vi "reseter.vi"(7 "Mode":enum16{"Init", "Set", "Get"}(ring)=enum."Get", 8 "Error In":errorcluster, 11 "Value":bool) -> (0 "Error Out":errorcluster, 3 "Value":bool)   [LabVIEW 2016]
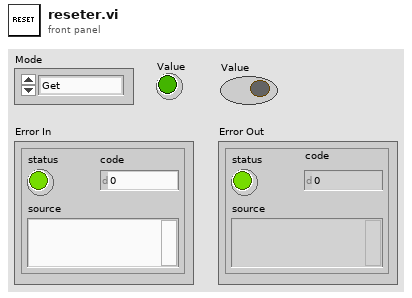
[diagram p1: front panel]
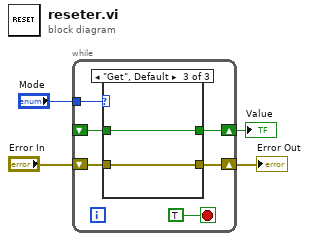
[diagram p0: block diagram]
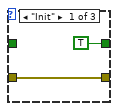
[diagram p2: hidden frame]
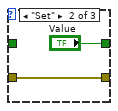
[diagram p3: hidden frame]
diagram:
  n1 = while {
    tunnel: "Mode" -> [w9]
    shift-right: [w7] -> w2
    shift-left: "Error In" -> [w8]
    shift-right: [w6] -> w1
    shift-left: _ -> [w5]
    stop <- TRUE stop-if-true
    n2 = case shown="\"Get\", Default" w9 {
      tunnel: w8 -> [w12 w13 w15]
      tunnel: [w12 w13 w15] -> w7
      tunnel: [TRUE "Value" w16] -> w6
      tunnel: w5 -> [_ _ w16]
      frame "Init" {
      }
      frame "Set" {
      }
      frame "Get", Default {
      }
    }
  }
  "Error Out" <- w2
  "Value" <- w1
